vi "ex_ParseMColPHeadLine.vi"(7 "delimiter":string, 8 "error in (no error)":errorcluster, 9 "channels":i32, 10 "file_params":T1={"include col headings?"=TRUE, "x_columns"=0, "col headings always?"=TRUE, "time preference"=0, "hide col headings"=FALSE} {"time preference" items=["Absolute", "Relative"]; "x_columns" items=["None", "One", "Multiple"]}, 11 "line":string) -> (0 "error out":errorcluster, 3 "elements":string[](array[string]))   [LabVIEW 2020]
uses:
  <vilib>/express/express input/ExFileReadBlock.llb/ex_ReadFileParams.ctl
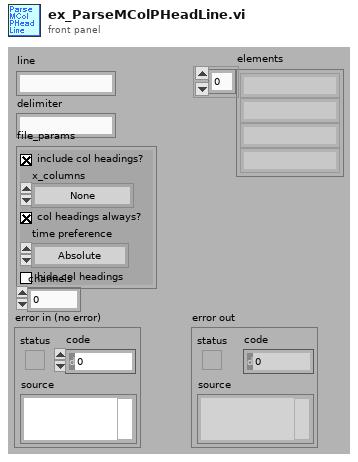
[diagram p1: front panel]
types:
  T1 = typedef "ex_ReadFileParams.ctl" = cluster{"include col headings?":bool, "x_columns":u16, "col headings always?":bool, "time preference":u16, "hide col headings":bool}
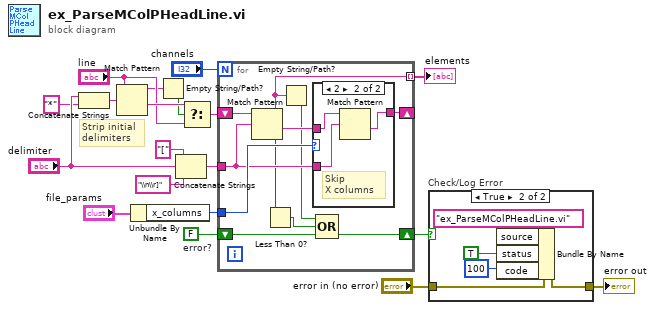
[diagram p0: block diagram]
diagram:
  w9 = FALSE  # error?
  # "Strip initial\ndelimiters"
  n1 = Concatenate Strings("delimiter", "*" ("string")) -> (w5:string)
  n2 = Match Pattern(string="line", regular expression=w5) -> (before substring=w2:string, after substring=w19:string)  [unwired: 3 out]
  n3 = Unbundle By Name("file_params") -> ("x_columns"=w11:u16)
  n4 = Empty String/Path?(string/path=w2) -> (empty?=w1:bool)
  n5 = Concatenate Strings("[", "delimiter", "\\n\\r]") -> (w14:string)
  n6 = Select(t=w19, s=w1, f="line") -> (s? t:f=w15:string)
  n7 = for {
    N: "channels" -> [_]
    shift-right: [w26] -> _
    shift-left: w15 -> [w30]
    tunnel: w14 -> [w27]
    tunnel: [w21] -> w10 mode=indexing
    tunnel: w11 -> [w29]
    shift-right: [w22] -> w8
    shift-left: w9 -> [w25]
    n8 = Match Pattern(string=w30, regular expression=w27) -> (before substring=w21:string, after substring=w28:string, offset past match=w23:i32)  [unwired: 2 out]
    n9 = Less Than 0?(x=w23) -> (x < 0?=w24:bool)
    n10 = Empty String/Path?(string/path=w21) -> (empty?=w20:bool)
    n11 = case shown="2" w29 {
      tunnel: w28 -> [w31 w34]
      tunnel: w27 -> [_ w33]
      tunnel: [w31 w32] -> w26
      frame Default {
        # "No X\ncolumns"
      }
      frame 2 {
        # "Skip\nX columns"
        n12 = Match Pattern(string=w34, regular expression=w33) -> (after substring=w32:string)  [unwired: 4 out]
      }
    }
    n13 = Compound Arithmetic op=OR(w20, w24, w25) -> (w22:bool)
  }
  "elements" <- w10
  n14 = case "Check/Log Error" shown="True" w8 {
    tunnel: "error in (no error)" -> [w35 w40]
    tunnel: [w35 w36] -> w6
    frame False {
    }
    frame True {
      n15 = Bundle By Name(cluster=w40, "source"="ex_ParseMColPHeadLine.vi", "status"=TRUE, "code"=100) -> (w36:errorcluster)
    }
  }
  "error out" <- w6
